vi "Part 1.vi"(11 "Input":string) -> (3 "Output":i64)   [LabVIEW 2021]
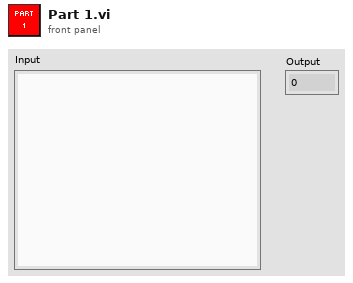
[diagram p1: front panel]
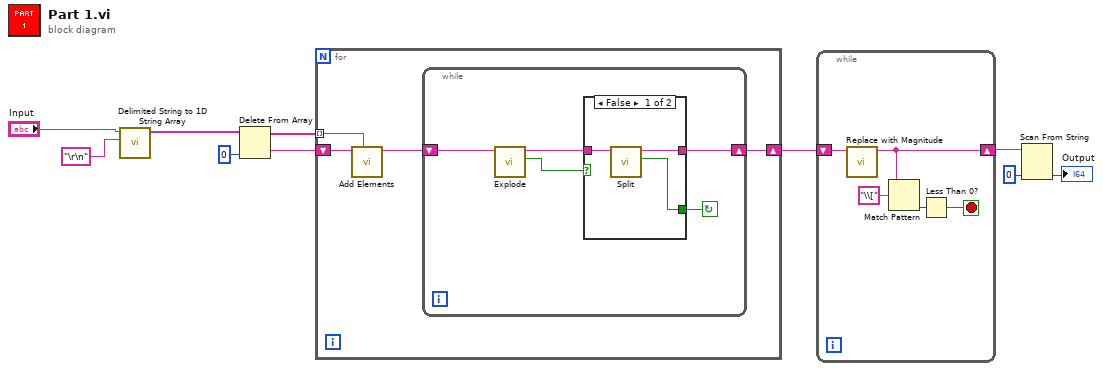
[diagram p0: block diagram]
diagram:
  n1 = call <vilib>:"Delimited String to 1D String Array.vi"("delimiter"="\r\n", "delimited string"="Input") -> ("string array"=w8:string[])  [unwired: 9 in]
  n2 = Delete From Array(array=w8, index=0) -> (deleted portion=w6:string, array with subset deleted=w5:string[])  [unwired: 1 in]
  n3 = for {
    shift-right: [w12] -> w4
    shift-left: w6 -> [w14]
    tunnel: w5 -> [w13] mode=indexing
    n4 = call "Add Elements.vi"("Element 2"=w13, "Element 1"=w14) -> ("Sum"=w11:string)  [unwired: 9 in]
    n5 = while {
      shift-right: [w19] -> w12
      shift-left: w11 -> [w17]
      stop <- w18 continue-if-true
      n6 = call "Explode.vi"("String In"=w17) -> ("Exploded?"=w15:bool, "String Out"=w16:string)  [unwired: 9 in]
      n7 = case shown="False" w15 {
        selector: w15 -> [_ w24]
        tunnel: [w22 w23] -> w19
        tunnel: [w21 w24] -> w18
        tunnel: w16 -> [w20 w23]
        frame False {
          n8 = call "Split.vi"("String In"=w20) -> ("Splitted?"=w21:bool, "String Out"=w22:string)  [unwired: 9 in]
        }
        frame True {
        }
      }
    }
  }
  n9 = while {
    shift-right: [w25] -> w3
    shift-left: w4 -> [w26]
    stop <- w27 stop-if-true
    n10 = call "Replace with Magnitude.vi"("String In"=w26) -> ("String Out"=w25:string)  [unwired: 10 in]
    n11 = Match Pattern(string=w25, regular expression="\\[") -> (offset past match=w28:i32)  [unwired: 1 in, 3 out]
    n12 = Less Than 0?(x=w28) -> (x < 0?=w27:bool)
  }
  n13 = Scan From String(input string=w3, default 1=i64 0 ("Output")) -> (output 1=→"Output":i64)  [unwired: 3 in, 3 out]
